vi "BigBen-01-16.vi"(0 "MethodenStartzeit":dbl, 1 "Methodenstart?":bool, 2 "Programmstart?":bool, 3 "Zykluslängen [s]":dbl[](array[numeric]), 4 "MethodenStartZyklusNummern":i32[](array[numeric])) -> (6 "MethodenStartzeit":dbl, 8 "ZyklusNummernGesamt":i32[](array[numeric]))   [LabVIEW 2017]
uses:
  <vilib>/functionblocks/Counter/Elapsed Timer/Elapsed Timer.vi
  GVZeitenZyklen.vi
  <vilib>/functionblocks/FB Core/FB Core.xnode
  <vilib>/functionblocks/NI_FunctionBlock Libraries.lvlib
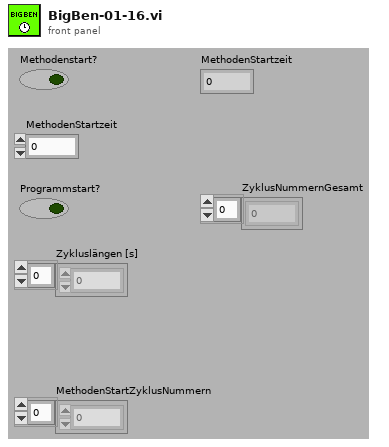
[diagram p1: front panel]
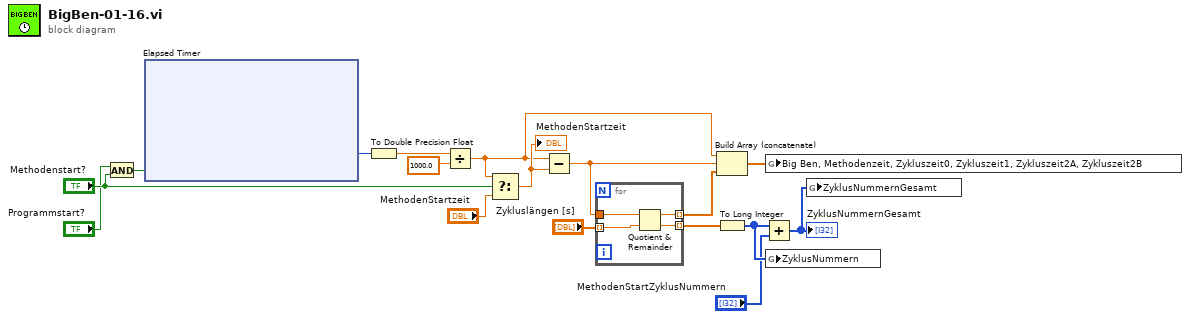
[diagram p0: block diagram]
diagram:
  n1 = And(x="Programmstart?", y="Methodenstart?") -> (x .and. y?=w4:bool)
  n2 = xnode "Elapsed Timer"("reset"=w4) -> ("elapsed time (ms)"=w1:i32)  [unwired: 2 in, 1 out]
  n3 = To Double Precision Float(number=w1) -> (double precision float=w2:dbl)
  n4 = Divide(x=w2, y=1000.0) -> (x/y=w16:dbl)
  n5 = Select(t=w16, s="Methodenstart?", f="MethodenStartzeit") -> (s? t:f=w17:dbl)
  "MethodenStartzeit" <- w17
  n6 = Subtract(x=w16, y=w17) -> (x-y=w8:dbl)
  n7 = for {
    tunnel: "Zykluslängen [s]" -> [w20] mode=indexing
    tunnel: w8 -> [w21]
    tunnel: [w19] -> w7 mode=indexing
    tunnel: [w18] -> w9 mode=indexing
    n8 = Quotient & Remainder(x=w21, y=w20) -> (x-y*floor(x/y)=w19:dbl, floor(x/y)=w18:dbl)
  }
  n9 = Build Array (concatenate)(w16, w8, w7) -> (w11:dbl[])
  n10 = To Long Integer(number=w9) -> (32bit integer=w12:i32[])
  n11 = Add(x=w12, y="MethodenStartZyklusNummern") -> (x+y=w13:i32[])
  "ZyklusNummernGesamt" <- w13
  n12 = global write "GVZeitenZyklen.vi" "Big Ben, Methodenzeit, Zykluszeit0, Zykluszeit1, Zykluszeit2A, Zykluszeit2B"(w11) -> ()
  n13 = global write "GVZeitenZyklen.vi" "ZyklusNummern"(w12) -> ()
  n14 = global write "GVZeitenZyklen.vi" "ZyklusNummernGesamt"(w13) -> ()
